vi "Untitled 2.vi"() -> ()   [LabVIEW 2020]
uses:
  <vilib>/express/express analysis/Spectral/Block/exnSpectralBlock spectral measurements peak poly.vi
  <vilib>/express/express analysis/Spectral/Block/exnSpectralBlock spectral measurements peak WFM.vi
  <vilib>/express/express analysis/Spectral/XNode/ExpressSpectralMeasurementsBlockNode.xnode
  <vilib>/measure/NI_MABase.lvlib
panel:
  out "Waveform Graph 2":waveform(dbl)(graph)
  out "Waveform Graph":dynamicdata(graph)
  out "Tw : frequency resoluton":dbl format="%#_4g"
  in  "N":dbl
  in  "fs":dbl
  in  "freq":dbl
  in  "amp":dbl
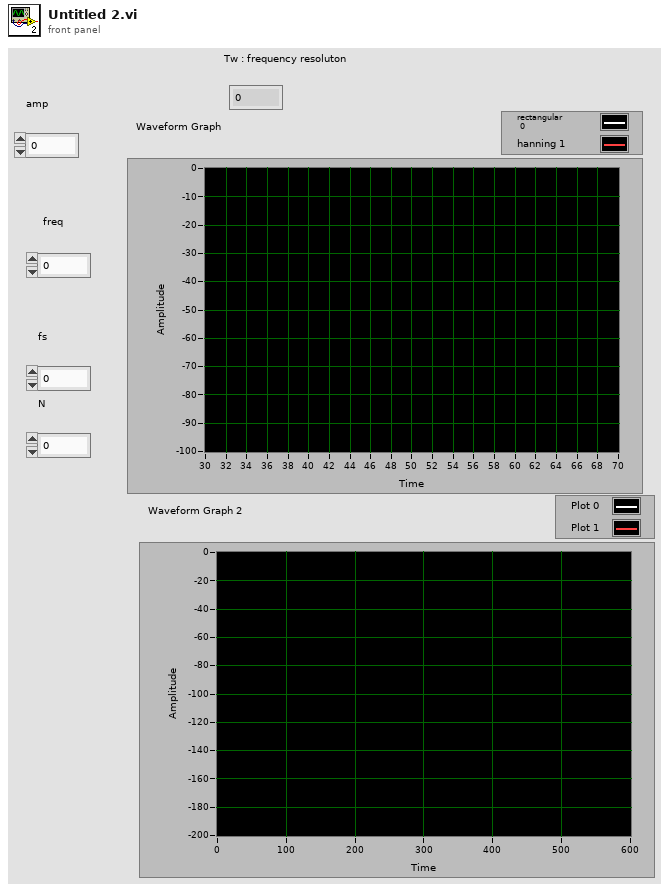
[diagram p1: front panel]
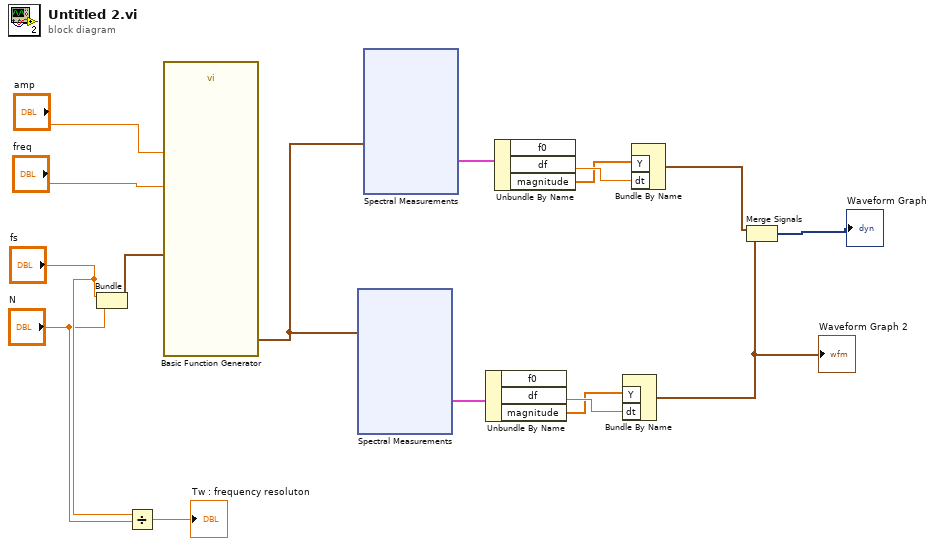
[diagram p0: block diagram]
diagram:
  n1 = Bundle("fs"="fs", "N"="N") -> (w16:cluster{"fs":dbl, "N":dbl})  [unwired: 1 in]
  n2 = Divide(x="fs", y="N") -> (x/y=→"Tw : frequency resoluton":dbl)
  n3 = call <vilib>:"Basic Function Generator.vi"("sampling info"=w16, "amplitude"="amp", "frequency"="freq") -> ("signal out"=w3:waveform(dbl))  [unwired: 6 in, 2 out]
  n4 = xnode "Spectral Measurements"("Signals"=w3) -> ("FFT - (Peak)"=w5:cluster{"f0":dbl, "df":dbl, "magnitude":dbl[]})  [unwired: 1 in, 2 out]
  n5 = xnode "Spectral Measurements"("Signals"=w3) -> ("FFT - (Peak)"=w10:cluster{"f0":dbl, "df":dbl, "magnitude":dbl[]})  [unwired: 1 in, 2 out]
  n6 = Unbundle By Name(w5) -> ("df"=w7:dbl, "magnitude"=w6:dbl[])  [unwired: 1 out]
  n7 = Unbundle By Name(w10) -> ("df"=w9:dbl, "magnitude"=w8:dbl[])  [unwired: 1 out]
  n8 = Bundle By Name("Y"=w6, "dt"=w7) -> (w1:waveform(dbl))  [unwired: 1 in]
  "Waveform Graph 2" <- w1
  n9 = Bundle By Name("Y"=w8, "dt"=w9) -> (w4:waveform(dbl))  [unwired: 1 in]
  n10 = Merge Signals "Merge Signals"(w4, w1) -> (→"Waveform Graph":dynamicdata)
